vi "RegisteredMsgUpdate.vi"(8 "error in (no error)":errorcluster, 10 "Msgs":refnum<class "MailBoxMessage.lvclass">[](array[class]), 11 "MC-ExternClient in":refnum<class "MC-ExternClient.lvclass">) -> (0 "error out":errorcluster, 3 "MC-ExternClient out":refnum<class "MC-ExternClient.lvclass">)   [LabVIEW 2020, in "MC-ExternClient.lvlib" / "MC-ExternClient.lvclass"]
uses:
  MC-ExternClient.lvclass
  MailboxManager/MailBoxMessage/MailBoxMessage.lvclass
  MC-ExternClientInterface/MC-ExternClientInterface.lvclass
  MC-ExternClient.lvclass/MC-ExternClient.ctl
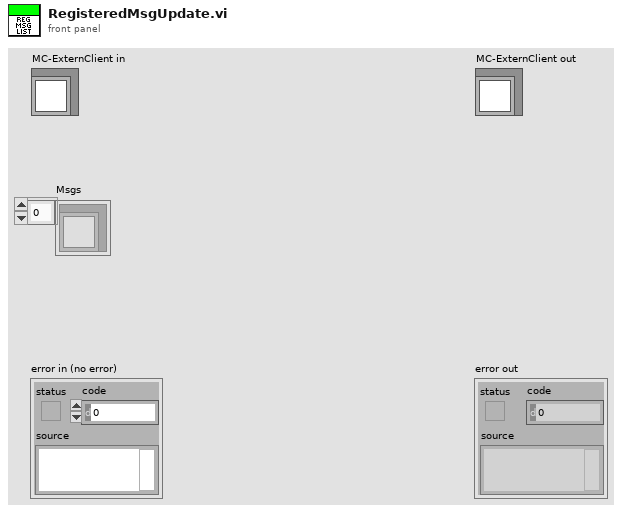
[diagram p1: front panel]
types:
  T1 = map{string, refnum<class "MailBoxMessage.lvclass">}
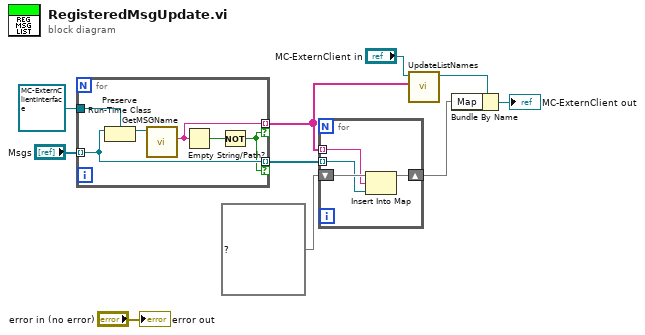
[diagram p0: block diagram]
diagram:
  n1 = for {
    tunnel: refnum<class "MC-ExternClientInterface.lvclass"> refnum ("MC-ExternClient.lvlib:MC-ExternClientInterface.lvclass") -> [w16]
    tunnel: "Msgs" -> [w12] mode=indexing
    tunnel: [w14] -> w5 mode=indexing if=w11
    tunnel: [w12] -> w4 mode=indexing if=w11
    n2 = Preserve Run-Time Class(object in=w12, 2:w16) -> (object out=w15:refnum<class "MC-ExternClientInterface.lvclass">)  [unwired: 1 in, 1 out]
    n3 = call-dynamic "GetMSGName.vi"("MC-ExternClientInterface in"=w15) -> ("NAME"=w14:string)  [unwired: 9 in, 1 out]
    n4 = Empty String/Path?(string/path=w14) -> (empty?=w13:bool)
    n5 = Not(x=w13) -> (.not. x?=w11:bool)
  }
  n6 = for {
    tunnel: w5 -> [w18] mode=indexing
    tunnel: w4 -> [w17] mode=indexing
    shift-right: [w19] -> w1
    shift-left: T1 {} ("Map") -> [w20]
    n7 = Insert Into Map(map in=w20, key=w18, value=w17) -> (map out=w19:T1)  [unwired: 2 out]
  }
  n8 = call-dynamic "UpdateListNames.vi"("Item Names"=w5, "MC-ExternClient in"="MC-ExternClient in") -> ("MC-ExternClient out"=w8:refnum<class "MC-ExternClient.lvclass">)  [unwired: 8 in, 1 out]
  n9 = Bundle By Name(cluster=w8, "Map"=w1) -> (→"MC-ExternClient out":refnum<class "MC-ExternClient.lvclass">)
  "error out" <- "error in (no error)"
